vi "Initialize and Register Sessions.vi"(8 "error in":errorcluster, 11 "sequence context in":refnum<k7>) -> (0 "error out":errorcluster)   [LabVIEW 2021, in "DmmMeasurementHAL.lvlib"]
uses:
  DmmMeasurementHAL.lvlib
  <vilib>/gRPC/Generated APIs/ni/measurementlink/sessionmanagement/v1/RPC Messages/ni_measurementlink_PinMapContext.ctl
  <vilib>/Plug-In SDKs/Clients/Session Management V1/Session Reservation/Session Reservation.lvclass/Session Reservation.ctl
  <vilib>/Plug-In SDKs/Clients/Session Management V1/Session Reservation/Initialize and Close Session Behavior.ctl
  <vilib>/Plug-In SDKs/Clients/Session Management V1/Session Reservation/Merge Invalid DVR Error.vi
  <vilib>/Plug-In SDKs/Clients/Session Management V1/Session Reservation/Is DVR Valid.vi
  <vilib>/Plug-In SDKs/Measurements/Helpers/Error Strings Global Internal.vi
  <vilib>/Utility/error.llb/Error Cluster From Error Code.vi
  HAL/Instruments/DMM_Base/DMM_Base.lvclass
  <vilib>/Plug-In SDKs/Clients/Session Management V1/Session Reservation/Session Reservation.lvclass
  HAL/Reusables/Get Pin Information.lvlib
  <vilib>/Plug-In SDKs/TestStand/NI Pin Map TestStand.lvlib
  <vilib>/gRPC/Generated APIs/ni/measurementlink/sessionmanagement/v1/ni.measurementlink.sessionmanagement.v1.api.lvlib
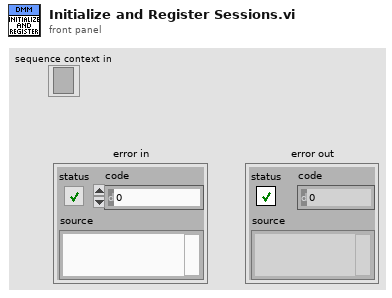
[diagram p1: front panel]
types:
  T1 = typedef "ni.measurementlink.sessionmanagement.v1.api.lvlib/ni_measurementlink_PinMapContext.ctl" = cluster{"pin_map_id":string, "sites":i32[]}
  T2 = typedef "ni.measurementlink.sessionmanagement.v1.api.lvlib/ni_measurementlink_sessionmanagement_v1_SessionInformation.ctl" = cluster{"session":T3, "resource_name":string, "channel_list":string, "instrument_type_id":string, "session_exists":bool, "channel_mappings":T4[]}
  T3 = typedef "ni.measurementlink.sessionmanagement.v1.api.lvlib/nidevice_grpc_Session.ctl" = cluster{"name":string}
  T4 = typedef "ni.measurementlink.sessionmanagement.v1.api.lvlib/ni_measurementlink_sessionmanagement_v1_ChannelMapping.ctl" = cluster{"pin_or_relay_name":string, "site":i32, "channel":string, "multiplexer_resource_name":string, "multiplexer_route":string}
  T5 = typedef "NI Session Management V1 Client.lvlib/Session Reservation.lvclass/Initialize and Close Session Behavior.ctl" = enum16{"Auto", "Initialize and Close", "Attach and Detach", "Initialize and Detach", "Attach and Close"}
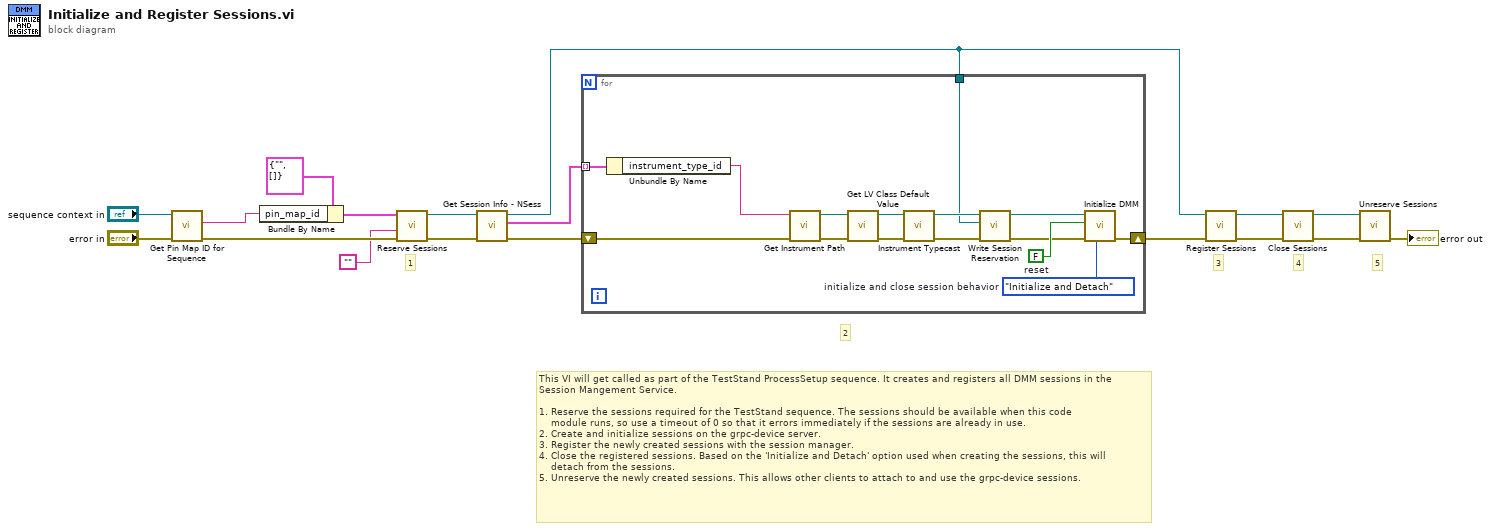
[diagram p0: block diagram]
diagram:
  # "This VI will get called as part of the TestStand ProcessSetup sequence. It creates and registers all DMM sessions in the\nSession Mangement Service.\n\n1. Reserve the sessions required for the TestStand sequence. The sessions should be available when this code\n    module runs, so use a timeout of 0 so that it errors immediately if the sessions are already in use.  \n2. Create and initialize sessions on the grpc-device server.\n3. Register the newly created sessions with the session manager.\n4. Close the registered sessions. Based on the 'Initialize and Detach' option used when creating the sessions, this will\n    detach from the sessions.\n5. Unreserve the newly created sessions. This allows other clients to attach to and use the grpc-device sessions."
  # "5"
  # "4"
  # "3"
  # "2"
  # "1"
  n1 = call <vilib>:"Get Pin Map ID for Sequence.vi"("error in"="error in", "sequence context in"="sequence context in") -> ("error out"=w16:errorcluster, "pin map id"=w15:string)  [unwired: 7 in, 1 out]
  n2 = Bundle By Name(cluster=T1 {"pin_map_id"="", "sites"=[]} ("pin map context"), "pin_map_id"=w15) -> (w1:T1)
  n3 = call <vilib>:"Reserve Sessions.vi"("error in"=w16, "instrument type id"="", "pin map context"=w1) -> ("error out"=w11:errorcluster, "session reservation out"=w10:refnum<class "Session Reservation.lvclass">)  [unwired: 7 in]
  n4 = call <vilib>:"Get Session Info - NSess .vi"("error in"=w11, "session reservation in"=w10) -> ("error out"=w13:errorcluster, "sessions info"=w12:T2[], "session reservation out"=w3:refnum<class "Session Reservation.lvclass">)  [unwired: 7 in]
  n5 = for {
    shift-right: [w30] -> w7
    shift-left: w13 -> [w22]
    tunnel: w12 -> [w33] mode=indexing
    tunnel: w3 -> [w23]
    w28 = FALSE  # reset
    w29 = Initialize_and_Close_Session_Behavior."Initialize and Detach"  # initialize and close session behavior
    n6 = Unbundle By Name(w33) -> ("instrument_type_id"=w20:string)
    n7 = call "Get Instrument Path.vi"("error in"=w22, "instrument_type_id"=w20) -> ("error out"=w21:errorcluster, "Instrument Path"=w19:path)  [unwired: 8 in]
    n8 = call <vilib>:"Get LV Class Default Value.vi"("error in (no error)"=w21, "class path"=w19) -> ("error out"=w32:errorcluster, "object"=w31:refnum<class>)  [unwired: 8 in]
    n9 = call "Instrument Typecast.vi"("error in (no error)"=w32, "pin instrument"=w31) -> ("error out"=w27:errorcluster, "instrument object"=w24:refnum<class "DMM_Base.lvclass">)  [unwired: 8 in]
    n10 = call-dynamic "Write Session Reservation.vi"("error in (no error)"=w27, "Session Reservation"=w23, "DMM_Base in"=w24) -> ("error out"=w26:errorcluster, "DMM_Base out"=w25:refnum<class "DMM_Base.lvclass">)  [unwired: 7 in]
    n11 = call-dynamic "Initialize DMM.vi"("initialize and close session behavior"=w29, "error in (no error)"=w26, "reset"=w28, "DMM_Base in"=w25) -> ("error out"=w30:errorcluster)  [unwired: 6 in, 1 out]
  }
  n12 = call <vilib>:"Register Sessions.vi"("error in"=w7, "session reservation in"=w3) -> ("error out"=w6:errorcluster, "session reservation out"=w8:refnum<class "Session Reservation.lvclass">)  [unwired: 8 in]
  n13 = call <vilib>:"Close Sessions.vi"("error in"=w6, "session reservation in"=w8) -> ("error out"=w5:errorcluster, "session reservation out"=w9:refnum<class "Session Reservation.lvclass">)  [unwired: 8 in]
  n14 = call <vilib>:"Unreserve Sessions.vi"("error in"=w5, "session reservation in"=w9) -> ("error out"=→"error out":errorcluster)  [unwired: 9 in]
